vi "Adaptive Echo Cancellation.vi"() -> ()   [LabVIEW 2019]
doc: "This example demonstrates how to apply a normalized LMS adaptive filter to adaptive echo cancellation applications. To remove echo from a sound signal, you must acquire the echo signal and the original clean sound signal that does not have echo. For the original clean sound, this example simulates it with a waveform file. For the echo signal, this example simulates it by applying an FIR filter to the waveform file. The FIR filter simulates the room impulse response, which is a linear system h(n) that models the room acoustic characters, including reverberation, resonance and reflections caused by the boundaries of the room and the objects in it.\n \nComplete the following steps to use this example.\n\n1. Display the <b>Adaptive Echo Cancellation</b> page and run the VI.\n\n2. Click the <b>Open Wave File</b> button to select a .wav file.\n\n3. Observe the <b>A. Original Sound</b>, <b>B. Echoes</b> and <b>C. Before Echo Cancellation = A + B2</b> graphs. You also can click the <b>Play</b> button on the top right of each graph to play the sound.\n\n4. Click the <b>Apply Echo Cancellation</b> button to remove the echo.\n\n5. Observe the <b>B. Echoes</b> graph, which displays the echo before and after you apply adaptive echo cancellation. The echo after adaptive echo cancellation is much smaller than the echo before adaptive echo cancellation.\n\n6. Observe the <b>D. After Echo Cancellation = A + B1</b> graph, which displays the resulting signal after adaptive echo cancellation."
uses:
  <vilib>/Analysis/3filter.llb/FIR Filter (DBL).vi
  <vilib>/addons/Adaptive Filters/Create/AFT Create FIR Normalized LMS (Real).vi
  <vilib>/addons/Adaptive Filters/Processing/AFT Filter Signal and Update Coefficients (Real, Array).vi
  <vilib>/Analysis/NI_AALBase.lvlib
  <vilib>/addons/Adaptive Filters/NI_AdaptiveFilter.lvlib
panel:
  in  "Tab Control":T1(tab)=enum."Adaptive Echo Cancellation"
  in  "Play Echo after AEC":bool
  in  "Play Echo":bool
  out "prompt 2":string="No wave file available,\nplease press \"Open wave file\""
  out "prompt":string="Applying echo cancellation, \nplease wait..."
  in  "Transmission Delay":dbl=0.3 min=0.0 max=0.001 step=5e-05 format="%#1.6f s"
  out "A. Original Sound":waveform(dbl)(graph)={"t0"=timestamp(0 s since 1904-01-01), "dt"=0.000125, "Y"=[]}
  out "D. After Echo Cancellation = A + B1":waveform(dbl)(graph)={"t0"=timestamp(0 s since 1904-01-01), "dt"=0.000125, "Y"=[]}
  in  "Filter Lecngth":i32=256
  out "C. Before Echo Cancellation = A + B2":waveform(dbl)(graph)={"t0"=timestamp(0 s since 1904-01-01), "dt"=0.000125, "Y"=[]}
  out "B. Echoes":waveform(dbl)[](graph)
  in  "Play Sound after AEC":bool
  in  "Open Wave File":bool
  in  "Apply Echo Cancellation":bool
  in  "Stop":bool
  in  "Step Size":dbl=0.1 min=0.0 max=1.0 step=0.05 format="%#1.6f"
  in  "Play Sound with Echo":bool
  in  "Play Original Sound":bool
  out "SNR after":dbl format="%#.2f dB"
  out "SNR before":dbl format="%#.2f dB"
  # "Refer to the Adaptive Echo Cancellation topic in the LabVIEW Help for more information about the background of adaptive echo cancellation. Select Help>>Show Context Help and move the cursor over the VI icon of this example for more information."
  # "SNR ="
  # "SNR ="
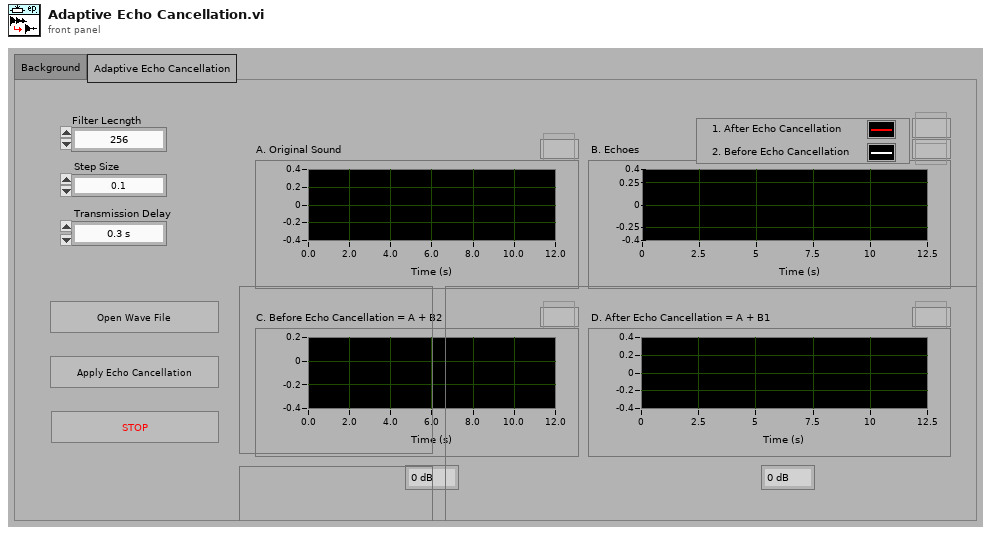
[diagram p1: front panel]
types:
  T1 = enum32{"Background", "Adaptive Echo Cancellation"}
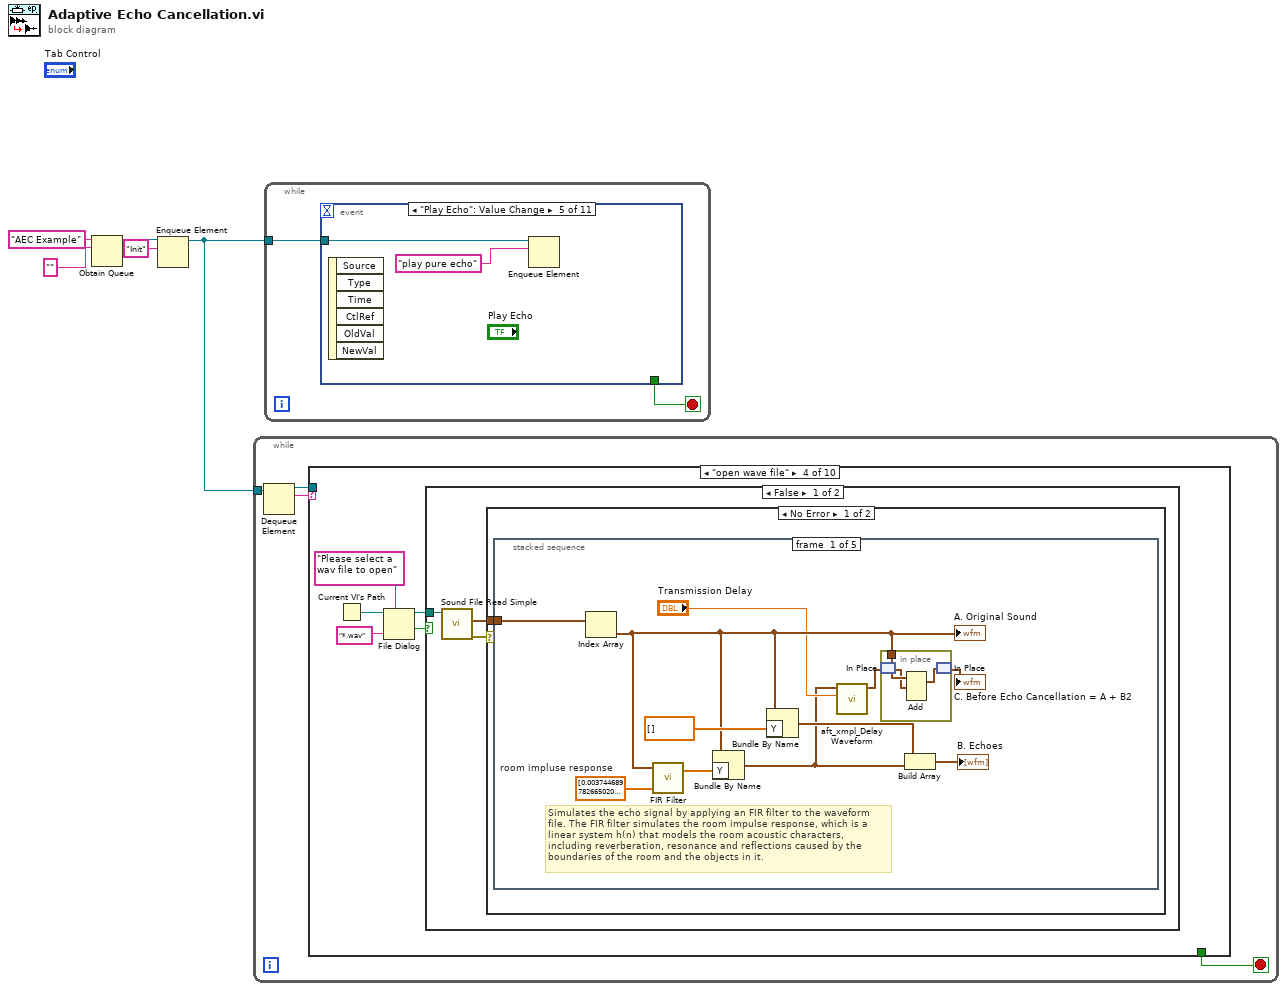
[diagram p0: block diagram]
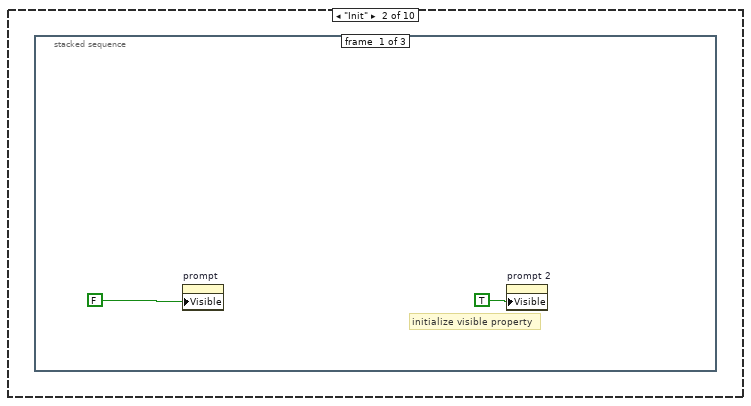
[diagram p3: hidden frame]
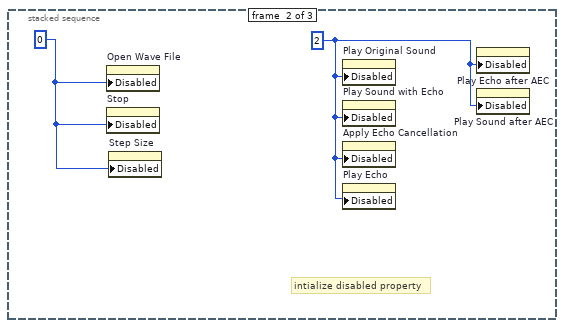
[diagram p4: hidden frame]
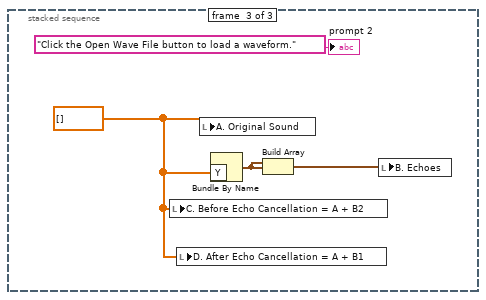
[diagram p5: hidden frame]
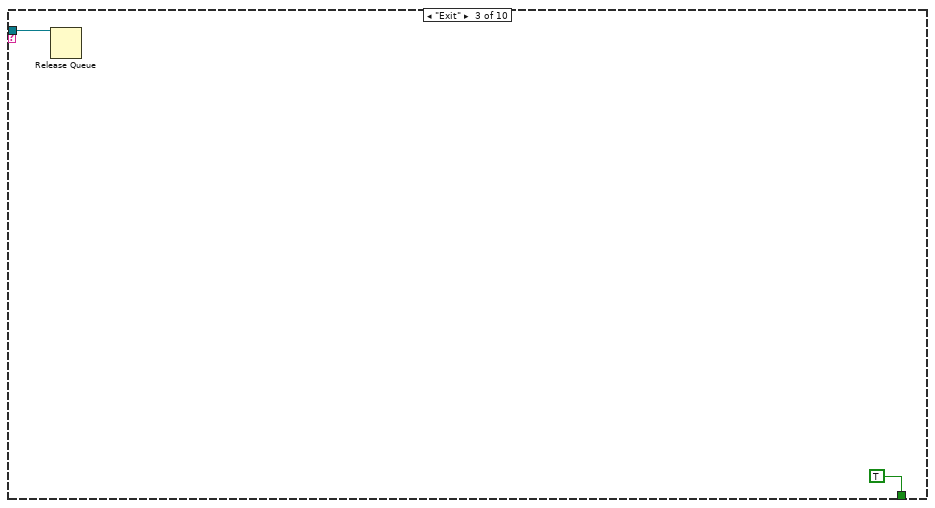
[diagram p6: hidden frame]
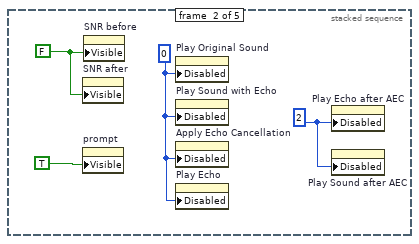
[diagram p7: hidden frame]
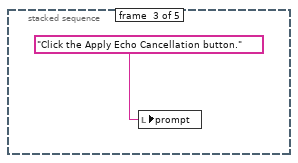
[diagram p8: hidden frame]
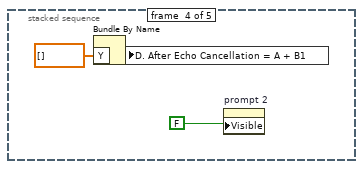
[diagram p9: hidden frame]
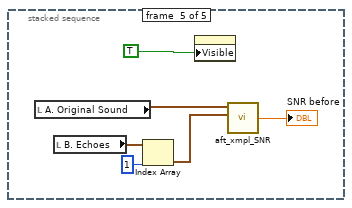
[diagram p10: hidden frame]
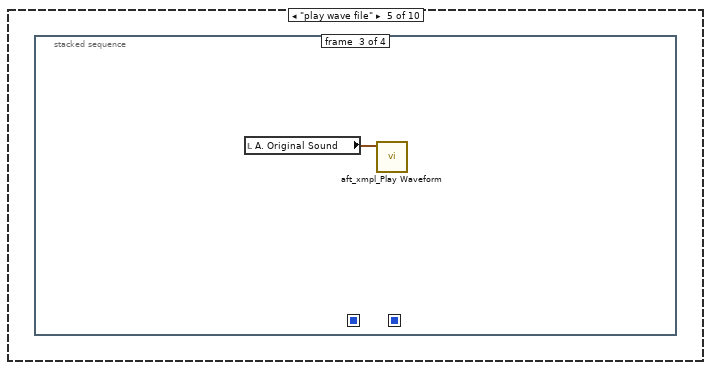
[diagram p13: hidden frame]
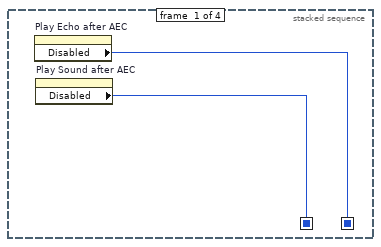
[diagram p14: hidden frame]
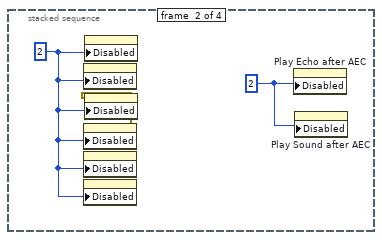
[diagram p15: hidden frame]
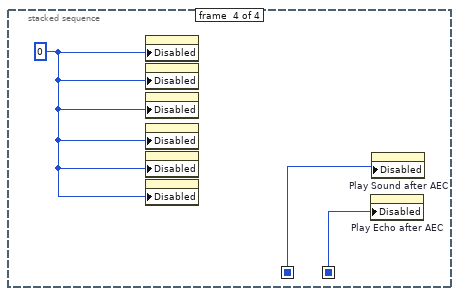
[diagram p16: hidden frame]
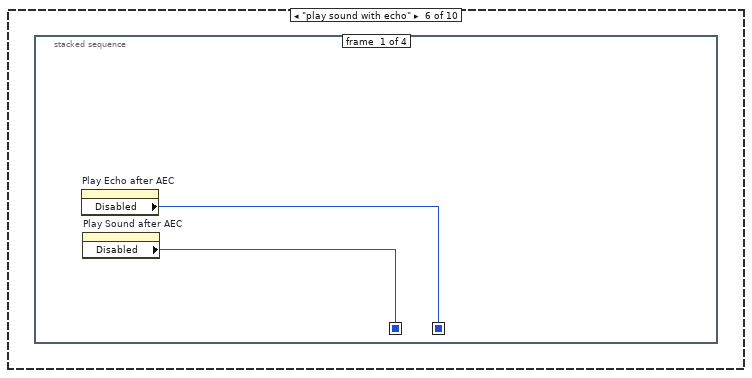
[diagram p17: hidden frame]
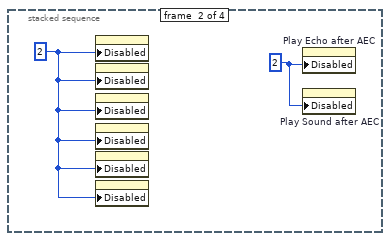
[diagram p18: hidden frame]
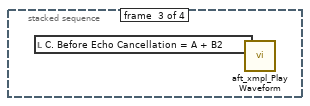
[diagram p19: hidden frame]
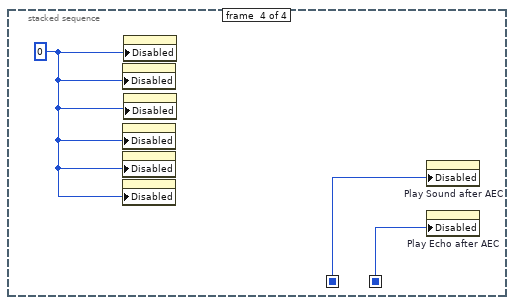
[diagram p20: hidden frame]
diagram:
  n1 = Obtain Queue(name (unnamed)="AEC Example", element data type="") -> (queue out=w3:refnum<queue>)  [unwired: 3 in, 2 out]
  n2 = Enqueue Element(queue=w3, element="Init") -> (queue out=w2:refnum<queue>)  [unwired: 1 in, 3 out]
  n3 = while {
    tunnel: w2 -> [w9]
    stop <- w6 stop-if-true
    n4 = Dequeue Element(queue=w9) -> (queue out=w7:refnum<queue>, element=w8:string)  [unwired: 1 in, 3 out]
    n5 = case shown="\"open wave file\"" w8 {
      tunnel: w7 -> [_ _ w19 _ _ _ _ _ _ _]
      tunnel: [_ _ TRUE _ _ _ _ _ _ _] -> w6
      frame "False", Default {
      }
      frame "Init" {
        n6 = stacked-sequence {
          frame #0 {
            # "initialize visible property"
            n7 = property on="prompt" class="Str"("Visible"=FALSE) -> ()  [unwired: 2 in, 2 out]
            n8 = property on="prompt 2" class="Str"("Visible"=TRUE) -> ()  [unwired: 2 in, 2 out]
          }
          frame #1 {
            w12 = u8 2 ("Disabled")
            w13 = u8 0 ("Disabled")
            # "intialize disabled property"
            n9 = property on="Open Wave File" class="Bool"("Disabled"=w13) -> ()  [unwired: 2 in, 2 out]
            n10 = property on="Stop" class="Bool"("Disabled"=w13) -> ()  [unwired: 2 in, 2 out]
            n11 = property on="Step Size" class="DigNum (strict)"("Disabled"=w13) -> ()  [unwired: 2 in, 2 out]
            n12 = property on="Play Original Sound" class="Bool"("Disabled"=w12) -> ()  [unwired: 2 in, 2 out]
            n13 = property on="Play Sound with Echo" class="Bool"("Disabled"=w12) -> ()  [unwired: 2 in, 2 out]
            n14 = property on="Apply Echo Cancellation" class="Bool"("Disabled"=w12) -> ()  [unwired: 2 in, 2 out]
            n15 = property on="Play Echo" class="Bool"("Disabled"=w12) -> ()  [unwired: 2 in, 2 out]
            n16 = property on="Play Echo after AEC" class="Bool"("Disabled"=w12) -> ()  [unwired: 2 in, 2 out]
            n17 = property on="Play Sound after AEC" class="Bool"("Disabled"=w12) -> ()  [unwired: 2 in, 2 out]
          }
          frame #2 {
            w16 = dbl[] []
            n18 = local write "C. Before Echo Cancellation = A + B2"(w16) -> ()
            n19 = local write "D. After Echo Cancellation = A + B1"(w16) -> ()
            n20 = local write "A. Original Sound"(w16) -> ()
            n21 = Bundle By Name("Y"=w16) -> (w15:waveform(dbl))  [unwired: 1 out]
            n22 = Build Array(w15, w15) -> (w14:waveform(dbl)[])
            n23 = local write "B. Echoes"(w14) -> ()
            "prompt 2" <- "Click the Open Wave File button to load a waveform." ("prompt 2")
          }
        }
      }
      frame "Exit" {
        n24 = Release Queue(queue=w19) -> ()  [unwired: 1 in, 4 out]
      }
      frame "open wave file" {
        n25 = Current VI's Path() -> (path=w24:path)
        n26 = File Dialog(6:"*.wav" ("pattern"), 7:"Please select a wav file to open" ("prompt"), 11:w24) -> (1:w23:bool, 3:w22:path)  [unwired: 1 in, 5 out]
        n27 = case shown="False" w23 {
          tunnel: w22 -> [w27 _]
          frame False {
            n28 = call <vilib>:"Sound File Read Simple.vi"("path"=w27) -> ("error out"=w25:errorcluster, "data"=w26:waveform(dbl)[])  [unwired: 4 in, 5 out]
            n29 = case shown="No Error" w25 {
              tunnel: w26 -> [w28 _]
              frame No Error {
                n30 = stacked-sequence {
                  tunnel: w28 -> [w39 _ _ _ _]
                  frame #0 {
                    w32 = dbl[] [0.0037446897826650203, 0.000973976512869415, 0.0034615532292998977, 0.011637172220574766, 4.5870634429664585e-05, -0.0034159836153683596, 0.0075052858689317135, 0.008372190560617483, 0.003385268774566946, 0.007845469277860001, 0.011566332481061073, 0.0038798372275538353, -0.005458129311006337, -0.0060413531526790605, -0.0017966244283888332, -0.0008714949457548632, -0.005920240906217639, -0.013389931971857675, -0.016741616497354672, -0.016039517409476213, -0.011445015823024748, -0.0028091145549090806, -0.0006459586952774438, -0.00550209743345678, -0.0058391788739494445, -0.0023574600102249355, 0.002755177145169217, 0.00831568148225722, 0.005325055796041635, -0.0018296761073409613, -0.0014307662041862397, -0.00016679196135441427, -0.007283331437230089, -0.01204210810208105, -0.006824697877890086, -0.0044702136461186575, -0.007381208093310558, -0.010126718211665615, -0.012866952548912543, -0.007710168040325809, -0.01692755086063684, -0.009491755843882439, -0.007613537193823553, -0.012033915056105052, 0.001447530035903867, -0.015148621737900693, -0.0011301872057858787, 0.1210377205355367, 0.1375140401938209, -0.013683280680633958, -0.09266747654191088, -0.06623951804519237, -0.025270412564893704, -0.0057463800851402305, -0.026986527829324803, -0.037052651044505766, -0.022134674943555564, -0.02561927652092903, -0.03703237399224595, -0.02361888473818607, 0.002803298034964096, 0.001446414990645078, -0.012546313552202785, -0.005676190450947756, 4.070283401402049e-05, 0.009654202804745523, 0.028352158954551492, 0.02575979558777393, 0.02296220303874006, 0.030695508350453416, 0.02182740677882357, 0.012929036842948497, 0.019862773204452566, 0.020878509708867198, 0.011489869142659096, 0.007505596969375783, 0.0064904351776687245, 0.0037416619339428856, 0.005137709453603007, 0.002893371918441247, -0.007710168040325809, -0.012866952548912543, -0.010126718211665615, -0.007381208093310558, -0.0044702136461186575, -0.006824697877890086, -0.01204210810208105, -0.007283331437230089, -0.00016679196135441427, -0.0014307662041862397, -0.0018296761073409613, 0.005325055796041635, 0.00831568148225722, 0.002755177145169217, -0.0023574600102249355, -0.0058391788739494445, -0.00550209743345678, -0.0006459586952774438, -0.0028091145549090806, -0.011445015823024748, -0.016039517409476213, -0.016741616497354672, -0.013389931971857675, -0.005920240906217639, -0.0008714949457548632, -0.0017966244283888332, -0.0060413531526790605, -0.005458129311006337, 0.0038798372275538353, 0.011566332481061073, 0.007845469277860001, 0.003385268774566946, 0.008372190560617483, 0.0075052858689317135, -0.0034159836153683596, 4.5870634429664585e-05, 0.011637172220574766, 0.0034615532292998977, 0.000973976512869415, 0.0037446897826650203]  # room impluse response
                    # "Simulates the echo signal by applying an FIR filter to the waveform file. The FIR filter simulates the room impulse response, which is a linear system h(n) that models the room acoustic characters, including reverberation, resonance and reflections caused by the boundaries of the room and the objects in it."
                    n31 = Index Array(array=w39) -> (element=w34:waveform(dbl))  [unwired: 1 in]
                    "A. Original Sound" <- w34
                    n32 = call-poly <vilib>:"FIR Filter.vi"("FIR Coefficients"=w32, "X"=w34) -> ("Filtered X"=w37:dbl[])  [unwired: 1 in, 2 out]
                    n33 = Bundle By Name(cluster=w34, "Y"=w37) -> (w30:waveform(dbl))
                    n34 = Bundle By Name(cluster=w34, "Y"=dbl[] []) -> (w33:waveform(dbl))
                    n35 = call "aft_xmpl_Delay Waveform.vi"("delay (sec)"="Transmission Delay", "input"=w30) -> ("output"=w29:waveform(dbl))  [unwired: 9 out]
                    n36 = in-place {
                      in-place-border: w34 -> [w41]
                      n37 = in-place-match #1(w29) -> (w40:waveform(dbl))
                      n38 = Add(1:w40, 2:w41) -> (0:w42:waveform(dbl))  [unwired: 1 in, 1 out]
                      n39 = in-place-match #1(w42) -> (→"C. Before Echo Cancellation = A + B2":waveform(dbl))
                    }
                    n40 = Build Array(w33, w30) -> (→"B. Echoes":waveform(dbl)[])
                  }
                  frame #1 {
                    w46 = FALSE ("Visible")
                    w43 = u8 2 ("Disabled")
                    w44 = u8 0 ("Disabled")
                    n41 = property on="SNR after" class="DigNum (strict)"("Visible"=w46) -> ()  [unwired: 2 in, 2 out]
                    n42 = property on="prompt" class="Str"("Visible"=TRUE) -> ()  [unwired: 2 in, 2 out]
                    n43 = property on="SNR before" class="DigNum (strict)"("Visible"=w46) -> ()  [unwired: 2 in, 2 out]
                    n44 = property on="Play Original Sound" class="Bool"("Disabled"=w44) -> ()  [unwired: 2 in, 2 out]
                    n45 = property on="Play Sound with Echo" class="Bool"("Disabled"=w44) -> ()  [unwired: 2 in, 2 out]
                    n46 = property on="Apply Echo Cancellation" class="Bool"("Disabled"=w44) -> ()  [unwired: 2 in, 2 out]
                    n47 = property on="Play Echo" class="Bool"("Disabled"=w44) -> ()  [unwired: 2 in, 2 out]
                    n48 = property on="Play Echo after AEC" class="Bool"("Disabled"=w43) -> ()  [unwired: 2 in, 2 out]
                    n49 = property on="Play Sound after AEC" class="Bool"("Disabled"=w43) -> ()  [unwired: 2 in, 2 out]
                  }
                  frame #2 {
                    n50 = local write "prompt"("Click the Apply Echo Cancellation button." ("prompt")) -> ()
                  }
                  frame #3 {
                    n51 = Bundle By Name("Y"=dbl[] []) -> (w48:waveform(dbl))  [unwired: 1 out]
                    n52 = local write "D. After Echo Cancellation = A + B1"(w48) -> ()
                    n53 = property on="prompt 2" class="Str"("Visible"=FALSE) -> ()  [unwired: 2 in, 2 out]
                  }
                  frame #4 {
                    n54 = local read "A. Original Sound"() -> (w55:waveform(dbl))
                    n55 = local read "B. Echoes"() -> (w54:waveform(dbl)[])
                    n56 = Index Array(array=w54, index=1) -> (element=w52:waveform(dbl))
                    n57 = property on="SNR before" class="DigNum (strict)"("Visible"=TRUE) -> ()  [unwired: 2 in, 2 out]
                    n58 = call "aft_xmpl_SNR.vi"("Signal"=w55, "Noise"=w52) -> ("snr"=→"SNR before":dbl)  [unwired: 3 out]
                  }
                }
              }
              frame Error {
              }
            }
          }
          frame True {
          }
        }
      }
      frame "play wave file" {
        n59 = stacked-sequence {
          seq-local: [w58 _ _ _] -> [_ _ _ w63]
          seq-local: [w57 _ _ _] -> [_ _ _ w64]
          frame #0 {
            n60 = property on="Play Echo after AEC" class="Bool"() -> ("Disabled"=w57:u8)  [unwired: 2 in, 2 out]
            n61 = property on="Play Sound after AEC" class="Bool"() -> ("Disabled"=w58:u8)  [unwired: 2 in, 2 out]
          }
          frame #1 {
            w59 = u8 2 ("Disabled")
            w60 = u8 2 ("Disabled")
            n62 = property on="Play Original Sound" class="Bool"("Disabled"=w60) -> ()  [unwired: 2 in, 2 out]
            n63 = property on="Play Sound with Echo" class="Bool"("Disabled"=w60) -> (error out=w61:errorcluster)  [unwired: 2 in, 1 out]
            n64 = property on="Apply Echo Cancellation" class="Bool"("Disabled"=w60) -> ()  [unwired: 2 in, 2 out]
            n65 = property on="Stop" class="Bool"("Disabled"=w60) -> ()  [unwired: 2 in, 2 out]
            n66 = property on="Open Wave File" class="Bool"("Disabled"=w60) -> ()  [unwired: 2 in, 2 out]
            n67 = property on="Play Echo" class="Bool"(error in=w61, "Disabled"=w60) -> ()  [unwired: 1 in, 2 out]
            n68 = property on="Play Echo after AEC" class="Bool"("Disabled"=w59) -> ()  [unwired: 2 in, 2 out]
            n69 = property on="Play Sound after AEC" class="Bool"("Disabled"=w59) -> ()  [unwired: 2 in, 2 out]
          }
          frame #2 {
            n70 = local read "A. Original Sound"() -> (w62:waveform(dbl))
            n71 = call "aft_xmpl_Play Waveform.vi"("sound"=w62) -> ()  [unwired: 11 out]
          }
          frame #3 {
            w65 = u8 0 ("Disabled")
            n72 = property on="Open Wave File" class="Bool"("Disabled"=w65) -> ()  [unwired: 2 in, 2 out]
            n73 = property on="Play Original Sound" class="Bool"("Disabled"=w65) -> ()  [unwired: 2 in, 2 out]
            n74 = property on="Play Echo" class="Bool"("Disabled"=w65) -> ()  [unwired: 2 in, 2 out]
            n75 = property on="Play Sound with Echo" class="Bool"("Disabled"=w65) -> ()  [unwired: 2 in, 2 out]
            n76 = property on="Apply Echo Cancellation" class="Bool"("Disabled"=w65) -> ()  [unwired: 2 in, 2 out]
            n77 = property on="Stop" class="Bool"("Disabled"=w65) -> ()  [unwired: 2 in, 2 out]
            n78 = property on="Play Echo after AEC" class="Bool"("Disabled"=w64) -> ()  [unwired: 2 in, 2 out]
            n79 = property on="Play Sound after AEC" class="Bool"("Disabled"=w63) -> ()  [unwired: 2 in, 2 out]
          }
        }
      }
      frame "play sound with echo" {
        n80 = stacked-sequence {
          seq-local: [w67 _ _ _] -> [_ _ _ w72]
          seq-local: [w66 _ _ _] -> [_ _ _ w71]
          frame #0 {
            n81 = property on="Play Echo after AEC" class="Bool"() -> ("Disabled"=w66:u8)  [unwired: 2 in, 2 out]
            n82 = property on="Play Sound after AEC" class="Bool"() -> ("Disabled"=w67:u8)  [unwired: 2 in, 2 out]
          }
          frame #1 {
            w68 = u8 2 ("Disabled")
            w69 = u8 2 ("Disabled")
            n83 = property on="Open Wave File" class="Bool"("Disabled"=w69) -> ()  [unwired: 2 in, 2 out]
            n84 = property on="Play Original Sound" class="Bool"("Disabled"=w69) -> ()  [unwired: 2 in, 2 out]
            n85 = property on="Play Echo" class="Bool"("Disabled"=w69) -> ()  [unwired: 2 in, 2 out]
            n86 = property on="Play Sound with Echo" class="Bool"("Disabled"=w69) -> ()  [unwired: 2 in, 2 out]
            n87 = property on="Apply Echo Cancellation" class="Bool"("Disabled"=w69) -> ()  [unwired: 2 in, 2 out]
            n88 = property on="Stop" class="Bool"("Disabled"=w69) -> ()  [unwired: 2 in, 2 out]
            n89 = property on="Play Echo after AEC" class="Bool"("Disabled"=w68) -> ()  [unwired: 2 in, 2 out]
            n90 = property on="Play Sound after AEC" class="Bool"("Disabled"=w68) -> ()  [unwired: 2 in, 2 out]
          }
          frame #2 {
            n91 = local read "C. Before Echo Cancellation = A + B2"() -> (w70:waveform(dbl))
            n92 = call "aft_xmpl_Play Waveform.vi"("sound"=w70) -> ()  [unwired: 11 out]
          }
          frame #3 {
            w73 = u8 0 ("Disabled")
            n93 = property on="Play Original Sound" class="Bool"("Disabled"=w73) -> ()  [unwired: 2 in, 2 out]
            n94 = property on="Play Sound with Echo" class="Bool"("Disabled"=w73) -> ()  [unwired: 2 in, 2 out]
            n95 = property on="Apply Echo Cancellation" class="Bool"("Disabled"=w73) -> ()  [unwired: 2 in, 2 out]
            n96 = property on="Stop" class="Bool"("Disabled"=w73) -> ()  [unwired: 2 in, 2 out]
            n97 = property on="Open Wave File" class="Bool"("Disabled"=w73) -> ()  [unwired: 2 in, 2 out]
            n98 = property on="Play Echo" class="Bool"("Disabled"=w73) -> ()  [unwired: 2 in, 2 out]
            n99 = property on="Play Sound after AEC" class="Bool"("Disabled"=w72) -> ()  [unwired: 2 in, 2 out]
            n100 = property on="Play Echo after AEC" class="Bool"("Disabled"=w71) -> ()  [unwired: 2 in, 2 out]
          }
        }
      }
      frame "play pure echo" {
        n101 = stacked-sequence {
          seq-local: [w75 _ _ _] -> [_ _ _ w82]
          seq-local: [w74 _ _ _] -> [_ _ _ w81]
          frame #0 {
            n102 = property on="Play Echo after AEC" class="Bool"() -> ("Disabled"=w74:u8)  [unwired: 2 in, 2 out]
            n103 = property on="Play Sound after AEC" class="Bool"() -> ("Disabled"=w75:u8)  [unwired: 2 in, 2 out]
          }
          frame #1 {
            w76 = u8 2 ("Disabled")
            w77 = u8 2 ("Disabled")
            n104 = property on="Open Wave File" class="Bool"("Disabled"=w77) -> ()  [unwired: 2 in, 2 out]
            n105 = property on="Play Original Sound" class="Bool"("Disabled"=w77) -> ()  [unwired: 2 in, 2 out]
            n106 = property on="Play Sound with Echo" class="Bool"("Disabled"=w77) -> ()  [unwired: 2 in, 2 out]
            n107 = property on="Apply Echo Cancellation" class="Bool"("Disabled"=w77) -> ()  [unwired: 2 in, 2 out]
            n108 = property on="Stop" class="Bool"("Disabled"=w77) -> ()  [unwired: 2 in, 2 out]
            n109 = property on="Play Echo" class="Bool"("Disabled"=w77) -> ()  [unwired: 2 in, 2 out]
            n110 = property on="Play Echo after AEC" class="Bool"("Disabled"=w76) -> ()  [unwired: 2 in, 2 out]
            n111 = property on="Play Sound after AEC" class="Bool"("Disabled"=w76) -> ()  [unwired: 2 in, 2 out]
          }
          frame #2 {
            n112 = local read "B. Echoes"() -> (w80:waveform(dbl)[])
            n113 = Index Array(array=w80, index=1) -> (element=w78:waveform(dbl))
            n114 = call "aft_xmpl_Play Waveform.vi"("sound"=w78) -> ()  [unwired: 11 out]
          }
          frame #3 {
            w83 = u8 0 ("Disabled")
            n115 = property on="Play Original Sound" class="Bool"("Disabled"=w83) -> ()  [unwired: 2 in, 2 out]
            n116 = property on="Play Sound with Echo" class="Bool"("Disabled"=w83) -> ()  [unwired: 2 in, 2 out]
            n117 = property on="Apply Echo Cancellation" class="Bool"("Disabled"=w83) -> ()  [unwired: 2 in, 2 out]
            n118 = property on="Stop" class="Bool"("Disabled"=w83) -> ()  [unwired: 2 in, 2 out]
            n119 = property on="Open Wave File" class="Bool"("Disabled"=w83) -> ()  [unwired: 2 in, 2 out]
            n120 = property on="Play Echo" class="Bool"("Disabled"=w83) -> ()  [unwired: 2 in, 2 out]
            n121 = property on="Play Echo after AEC" class="Bool"("Disabled"=w81) -> ()  [unwired: 2 in, 2 out]
            n122 = property on="Play Sound after AEC" class="Bool"("Disabled"=w82) -> ()  [unwired: 2 in, 2 out]
          }
        }
      }
      frame "echo cancelling" {
        n123 = stacked-sequence {
          frame #0 {
            w86 = u8 2 ("Disabled")
            n124 = property on="prompt" class="Str"("Visible"=TRUE) -> ()  [unwired: 2 in, 2 out]
            n125 = property on="Open Wave File" class="Bool"("Disabled"=w86) -> ()  [unwired: 2 in, 2 out]
            n126 = property on="Play Original Sound" class="Bool"("Disabled"=w86) -> ()  [unwired: 2 in, 2 out]
            n127 = property on="Play Echo" class="Bool"("Disabled"=w86) -> ()  [unwired: 2 in, 2 out]
            n128 = property on="Play Sound with Echo" class="Bool"("Disabled"=w86) -> ()  [unwired: 2 in, 2 out]
            n129 = property on="Apply Echo Cancellation" class="Bool"("Disabled"=w86) -> ()  [unwired: 2 in, 2 out]
            n130 = property on="Stop" class="Bool"("Disabled"=w86) -> ()  [unwired: 2 in, 2 out]
            n131 = property on="Play Sound after AEC" class="Bool"("Disabled"=w86) -> ()  [unwired: 2 in, 2 out]
            n132 = property on="Play Echo after AEC" class="Bool"("Disabled"=w86) -> ()  [unwired: 2 in, 2 out]
            n133 = property on="SNR after" class="DigNum (strict)"("Visible"=FALSE) -> ()  [unwired: 2 in, 2 out]
            n134 = property on="prompt" class="Str"("Visible"=TRUE) -> ()  [unwired: 2 in, 2 out]
            "prompt" <- "Applying echo cancellation, \nplease wait..." ("prompt")
          }
          frame #1 {
            n135 = local read "A. Original Sound"() -> (w101:waveform(dbl))
            n136 = local read "B. Echoes"() -> (w105:waveform(dbl)[])
            n137 = Unbundle By Name(w101) -> ("Y"=w95:dbl[])
            n138 = Index Array(array=w105, index=1) -> (element=w103:waveform(dbl))
            n139 = call-poly <vilib>:"AFT Create FIR Normalized LMS.vi"("step size"="Step Size", "filter length"="Filter Lecngth") -> ("error out"=w93:errorcluster, "adaptive filter out"=w90:refnum<k20>)  [unwired: 2 in, 6 out]
            n140 = Unbundle By Name(w103) -> ("Y"=w97:dbl[])
            n141 = call-poly <vilib>:"AFT Filter Signal and Update Coefficients.vi"("error in (no error)"=w93, "d(n)"=w97, "x(n)"=w95, "adaptive filter in"=w90) -> ("error out"=w92:errorcluster, "e(n)"=w94:dbl[], "adaptive filter out"=w107:refnum<k20>)  [unwired: 2 in, 3 out]
            n142 = local read "Transmission Delay"() -> (w99:dbl)
            n143 = Bundle By Name(cluster=w103, "Y"=w94) -> (w96:waveform(dbl))
            n144 = call <vilib>:"AFT Destroy Adaptive Filter.vi"("error in (no error)"=w92, "adaptive filter in"=w107) -> ("error out"=w89:errorcluster)  [unwired: 9 out]
            n145 = call "aft_xmpl_Delay Waveform.vi"("delay (sec)"=w99, "input"=w96) -> ("output"=w98:waveform(dbl))  [unwired: 9 out]
            n146 = in-place {
              in-place-border: w101 -> [w110]
              n147 = in-place-match #2(w98) -> (w108:waveform(dbl))
              n148 = Add(1:w108, 2:w110) -> (0:w109:waveform(dbl))  [unwired: 1 in, 1 out]
              n149 = in-place-match #2(w109) -> (→"D. After Echo Cancellation = A + B1":waveform(dbl))
            }
            n150 = call <vilib>:"Simple Error Handler.vi"("error in (no error)"=w89) -> ()  [unwired: 1 in, 8 out]
            n151 = Build Array(w96, w103) -> (w102:waveform(dbl)[])
            n152 = local write "B. Echoes"(w102) -> ()
          }
          frame #2 {
            w111 = u8 0 ("Disabled")
            n153 = property on="prompt" class="Str"("Visible"=FALSE) -> ()  [unwired: 2 in, 2 out]
            n154 = property on="Open Wave File" class="Bool"("Disabled"=w111) -> ()  [unwired: 2 in, 2 out]
            n155 = property on="Play Original Sound" class="Bool"("Disabled"=w111) -> ()  [unwired: 2 in, 2 out]
            n156 = property on="Play Sound with Echo" class="Bool"("Disabled"=w111) -> ()  [unwired: 2 in, 2 out]
            n157 = property on="Apply Echo Cancellation" class="Bool"("Disabled"=w111) -> ()  [unwired: 2 in, 2 out]
            n158 = property on="Stop" class="Bool"("Disabled"=w111) -> ()  [unwired: 2 in, 2 out]
            n159 = property on="Play Echo after AEC" class="Bool"("Disabled"=w111) -> ()  [unwired: 2 in, 2 out]
            n160 = property on="Play Echo" class="Bool"("Disabled"=w111) -> ()  [unwired: 2 in, 2 out]
            n161 = property on="Play Sound after AEC" class="Bool"("Disabled"=w111) -> ()  [unwired: 2 in, 2 out]
            n162 = property on="Step Size" class="DigNum (strict)"("Disabled"=u8 0) -> ()  [unwired: 2 in, 2 out]
          }
          frame #3 {
            n163 = local read "D. After Echo Cancellation = A + B1"() -> (w116:waveform(dbl))
            n164 = local read "A. Original Sound"() -> (w115:waveform(dbl))
            n165 = in-place {
              in-place-border: w115 -> [w120]
              n166 = in-place-match #3(w116) -> (w121:waveform(dbl))
              n167 = Subtract(1:w120, 2:w121) -> (0:w119:waveform(dbl))  [unwired: 1 in, 1 out]
              n168 = in-place-match #3(w119) -> (w114:waveform(dbl))
            }
            n169 = call "aft_xmpl_SNR.vi"("Signal"=w115, "Noise"=w114) -> ("snr"=→"SNR after":dbl)  [unwired: 3 out]
            n170 = property on="SNR after" class="DigNum (strict)"("Visible"=TRUE) -> ()  [unwired: 2 in, 2 out]
          }
        }
      }
      frame "play residual echo" {
        n171 = stacked-sequence {
          frame #0 {
            w122 = u8 2 ("Disabled")
            (unwired) TRUE ("Visible")
            w123 = u8 2 ("Disabled")
            n172 = property on="Play Original Sound" class="Bool"("Disabled"=w123) -> ()  [unwired: 2 in, 2 out]
            n173 = property on="Play Sound with Echo" class="Bool"("Disabled"=w123) -> ()  [unwired: 2 in, 2 out]
            n174 = property on="Apply Echo Cancellation" class="Bool"("Disabled"=w123) -> ()  [unwired: 2 in, 2 out]
            n175 = property on="Stop" class="Bool"("Disabled"=w123) -> ()  [unwired: 2 in, 2 out]
            n176 = property on="Open Wave File" class="Bool"("Disabled"=w123) -> ()  [unwired: 2 in, 2 out]
            n177 = property on="Play Echo" class="Bool"("Disabled"=w123) -> ()  [unwired: 2 in, 2 out]
            n178 = property on="Play Echo after AEC" class="Bool"("Disabled"=w122) -> ()  [unwired: 2 in, 2 out]
            n179 = property on="Play Sound after AEC" class="Bool"("Disabled"=w122) -> ()  [unwired: 2 in, 2 out]
          }
          frame #1 {
            n180 = local read "B. Echoes"() -> (w126:waveform(dbl)[])
            n181 = Index Array(array=w126, index=0) -> (element=w124:waveform(dbl))
            n182 = call "aft_xmpl_Play Waveform.vi"("sound"=w124) -> ()  [unwired: 11 out]
          }
          frame #2 {
            (unwired) FALSE ("Visible")
            w127 = u8 0 ("Disabled")
            n183 = property on="Play Original Sound" class="Bool"("Disabled"=w127) -> ()  [unwired: 2 in, 2 out]
            n184 = property on="Play Sound with Echo" class="Bool"("Disabled"=w127) -> ()  [unwired: 2 in, 2 out]
            n185 = property on="Apply Echo Cancellation" class="Bool"("Disabled"=w127) -> ()  [unwired: 2 in, 2 out]
            n186 = property on="Stop" class="Bool"("Disabled"=w127) -> ()  [unwired: 2 in, 2 out]
            n187 = property on="Play Echo after AEC" class="Bool"("Disabled"=w127) -> ()  [unwired: 2 in, 2 out]
            n188 = property on="Play Sound after AEC" class="Bool"("Disabled"=w127) -> ()  [unwired: 2 in, 2 out]
            n189 = property on="Open Wave File" class="Bool"("Disabled"=w127) -> ()  [unwired: 2 in, 2 out]
            n190 = property on="Play Echo" class="Bool"("Disabled"=w127) -> ()  [unwired: 2 in, 2 out]
          }
        }
      }
      frame "play sound with residual echo" {
        n191 = stacked-sequence {
          seq-local: [w128 _ _ _] -> [_ _ _ w134]
          seq-local: [w129 _ _ _] -> [_ _ _ w133]
          frame #0 {
            n192 = property on="Play Echo after AEC" class="Bool"() -> ("Disabled"=w128:u8)  [unwired: 2 in, 2 out]
            n193 = property on="Play Sound after AEC" class="Bool"() -> ("Disabled"=w129:u8)  [unwired: 2 in, 2 out]
          }
          frame #1 {
            w130 = u8 2 ("Disabled")
            w131 = u8 2 ("Disabled")
            n194 = property on="Play Original Sound" class="Bool"("Disabled"=w131) -> ()  [unwired: 2 in, 2 out]
            n195 = property on="Play Echo" class="Bool"("Disabled"=w131) -> ()  [unwired: 2 in, 2 out]
            n196 = property on="Play Sound with Echo" class="Bool"("Disabled"=w131) -> ()  [unwired: 2 in, 2 out]
            n197 = property on="Apply Echo Cancellation" class="Bool"("Disabled"=w131) -> ()  [unwired: 2 in, 2 out]
            n198 = property on="Stop" class="Bool"("Disabled"=w131) -> ()  [unwired: 2 in, 2 out]
            n199 = property on="Open Wave File" class="Bool"("Disabled"=w131) -> ()  [unwired: 2 in, 2 out]
            n200 = property on="Play Echo after AEC" class="Bool"("Disabled"=w130) -> ()  [unwired: 2 in, 2 out]
            n201 = property on="Play Sound after AEC" class="Bool"("Disabled"=w130) -> ()  [unwired: 2 in, 2 out]
          }
          frame #2 {
            n202 = local read "D. After Echo Cancellation = A + B1"() -> (w132:waveform(dbl))
            n203 = call "aft_xmpl_Play Waveform.vi"("sound"=w132) -> ()  [unwired: 11 out]
          }
          frame #3 {
            w135 = u8 0 ("Disabled")
            n204 = property on="Open Wave File" class="Bool"("Disabled"=w135) -> ()  [unwired: 2 in, 2 out]
            n205 = property on="Play Original Sound" class="Bool"("Disabled"=w135) -> ()  [unwired: 2 in, 2 out]
            n206 = property on="Play Echo" class="Bool"("Disabled"=w135) -> ()  [unwired: 2 in, 2 out]
            n207 = property on="Play Sound with Echo" class="Bool"("Disabled"=w135) -> ()  [unwired: 2 in, 2 out]
            n208 = property on="Apply Echo Cancellation" class="Bool"("Disabled"=w135) -> ()  [unwired: 2 in, 2 out]
            n209 = property on="Stop" class="Bool"("Disabled"=w135) -> ()  [unwired: 2 in, 2 out]
            n210 = property on="Play Echo after AEC" class="Bool"("Disabled"=w133) -> ()  [unwired: 2 in, 2 out]
            n211 = property on="Play Sound after AEC" class="Bool"("Disabled"=w134) -> ()  [unwired: 2 in, 2 out]
          }
        }
      }
    }
  }
  n212 = while {
    tunnel: w2 -> [w137]
    stop <- w136 stop-if-true
    n213 = event shown="[4] \"Play Echo\": Value Change" {
      selector: _ -> [_ _ _ _ _ _ _ _ _ _ _]
      dyn-events: _ -> [_ _ _ _ _ _ _ _ _ _ _]
      timeout: _ -> [_ _ _ _ _ _ _ _ _ _ _]
      tunnel: w137 -> [_ w139 w141 w143 w145 w147 w149 w151 _ _ w159]
      tunnel: [_ _ _ _ _ _ _ _ _ _ TRUE] -> w136
      event Timeout {
        n214 = event-data() -> ()  [unwired: 3 out]
      }
      event "Open Wave File": Value Change {
        n215 = event-data() -> ()  [unwired: 7 out]
        n216 = Enqueue Element(queue=w139, element="open wave file") -> ()  [unwired: 1 in, 4 out]
      }
      event "Play Original Sound": Value Change {
        n217 = event-data() -> ()  [unwired: 7 out]
        n218 = Enqueue Element(queue=w141, element="play wave file") -> ()  [unwired: 1 in, 4 out]
      }
      event "Play Sound with Echo": Value Change {
        n219 = event-data() -> ()  [unwired: 7 out]
        n220 = Enqueue Element(queue=w143, element="play sound with echo") -> ()  [unwired: 1 in, 4 out]
      }
      event "Play Echo": Value Change {
        n221 = event-data() -> ()  [unwired: 7 out]
        n222 = Enqueue Element(queue=w145, element="play pure echo") -> ()  [unwired: 1 in, 4 out]
      }
      event "Apply Echo Cancellation": Value Change {
        n223 = event-data() -> ()  [unwired: 7 out]
        n224 = Enqueue Element(queue=w147, element="echo cancelling") -> ()  [unwired: 1 in, 4 out]
      }
      event "Play Echo after AEC": Value Change {
        n225 = event-data() -> ()  [unwired: 7 out]
        n226 = Enqueue Element(queue=w149, element="play residual echo") -> ()  [unwired: 1 in, 4 out]
      }
      event "Play Sound after AEC": Value Change {
        n227 = event-data() -> ()  [unwired: 7 out]
        n228 = Enqueue Element(queue=w151, element="play sound with residual echo") -> ()  [unwired: 1 in, 4 out]
      }
      event "Transmission Delay": Value Change {
        n229 = event-data() -> ()  [unwired: 7 out]
        n230 = property on="SNR after" class="DigNum (strict)"("Visible"=FALSE) -> ()  [unwired: 2 in, 2 out]
        n231 = local write "prompt"("Echo property changed, press\n \"Apply echo cancellation\" to continue" ("prompt")) -> ()
        n232 = property on="prompt" class="Str"("Visible"=TRUE) -> ()  [unwired: 2 in, 2 out]
      }
      event "Filter Lecngth", "Step Size": Value Change {
        n233 = event-data() -> ()  [unwired: 7 out]
        n234 = local write "prompt"("Adaptive filter settings changed, press\n \"Apply echo cancellation\" to continue" ("prompt")) -> ()
        n235 = property on="prompt" class="Str"("Visible"=TRUE) -> ()  [unwired: 2 in, 2 out]
        n236 = property on="SNR after" class="DigNum (strict)"("Visible"=FALSE) -> ()  [unwired: 2 in, 2 out]
      }
      event "Stop": Value Change {
        n237 = event-data() -> ()  [unwired: 7 out]
        n238 = Enqueue Element(queue=w159, element="Exit") -> ()  [unwired: 1 in, 4 out]
      }
    }
  }
